vi "Destroy Events.vi"(8 "error in (no error)":errorcluster, 11 "NI Force Task in":refnum<class "NI Force Task.lvclass">) -> (0 "error out":errorcluster, 3 "NI Force Task out":refnum<class "NI Force Task.lvclass">)   [LabVIEW 2020, in "NI Force Task.lvlib" / "NI Force Task.lvclass"]
uses:
  NI Force Task.lvclass
  C:/Program Files/National Instruments/LabVIEW 2020/vi.lib/ActorFramework/Actor/Actor.lvclass
  <vilib>/ActorFramework/Actor/Actor.lvclass/Actor.ctl
  NI Force Task.lvclass/NI Force Task.ctl
  GUI Interface Messages/End Preview Msg/End Preview Msg.lvclass/End Preview Msg.ctl
  <vilib>/ActorFramework/Message Enqueuer/Message Enqueuer.lvclass/Message Enqueuer.ctl
  <vilib>/ActorFramework/Message Enqueuer/Enqueue.vi
  GUI Interface Messages/End Preview Msg/End Preview Msg.lvclass
  C:/Program Files/National Instruments/LabVIEW 2020/vi.lib/ActorFramework/Message/Message.lvclass
  <vilib>/ActorFramework/Stop Msg/Stop Msg.lvclass
  <vilib>/ActorFramework/Message Priority Queue/Priority Enqueue.vi
  <vilib>/ActorFramework/Actor/Actor.lvclass
panel:
  out "error out 2":errorcluster
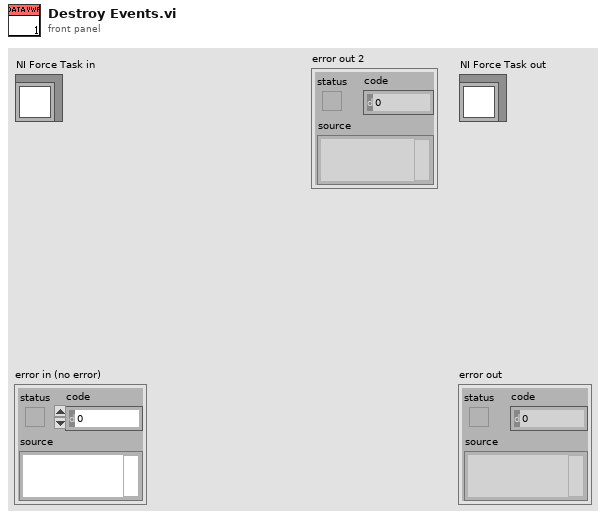
[diagram p1: front panel]
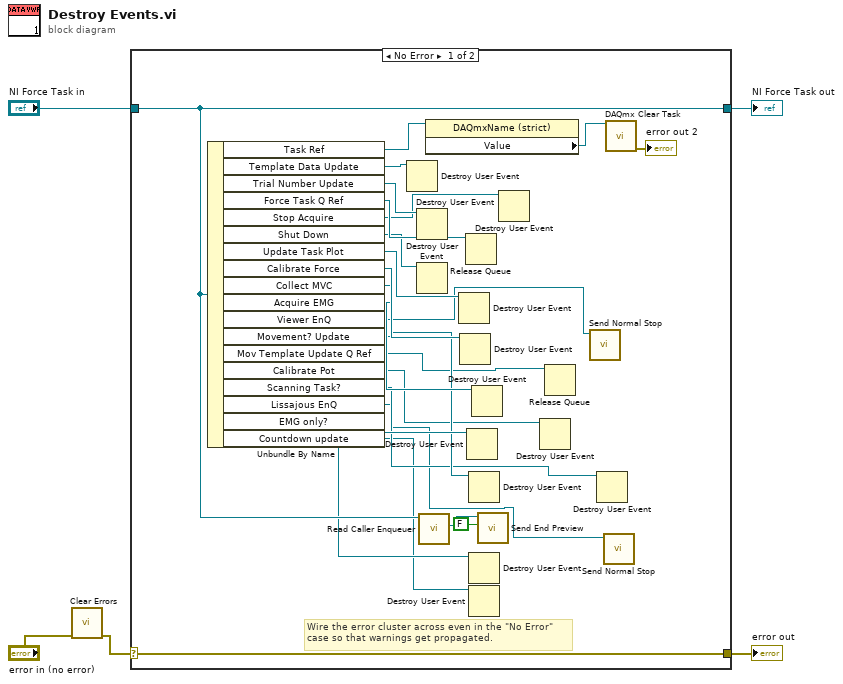
[diagram p0: block diagram]
diagram:
  n1 = call <vilib>:"Clear Errors.vi"("error in (no error)"="error in (no error)") -> ("error out"=w1:errorcluster)  [unwired: 5 in, 1 out]
  n2 = case shown="No Error" w1 {
    selector: w1 -> [w29 w31]
    tunnel: [w29 w31] -> w5
    tunnel: [w15 w30] -> w3
    tunnel: "NI Force Task in" -> [w15 w30]
    frame No Error {
      # "Wire the error cluster across even in the \"No Error\"\ncase so that warnings get propagated."
      n3 = Unbundle By Name(w15) -> ("Task Ref"=w22:refnum<vi>, "Template Data Update"=w28:refnum<user-event>, "Trial Number Update"=w27:refnum<user-event>, "Force Task Q Ref"=w26:refnum<queue>, "Stop Acquire"=w25:refnum<user-event>, "Shut Down"=w24:refnum<user-event>, "Update Task Plot"=w20:refnum<user-event>, "Calibrate Force"=w19:refnum<user-event>, "Collect MVC"=w18:refnum<user-event>, "Acquire EMG"=w17:refnum<user-event>, "Viewer EnQ"=w13:refnum<class "Message Enqueuer.lvclass">, "Movement? Update"=w12:refnum<user-event>, "Mov Template Update Q Ref"=w11:refnum<queue>, "Calibrate Pot"=w10:refnum<user-event>, "Scanning Task?"=w9:refnum<user-event>, "Lissajous EnQ"=w8:refnum<class "Message Enqueuer.lvclass">, "EMG only?"=w7:refnum<user-event>, "Countdown update"=w6:refnum<user-event>)
      n4 = Destroy User Event(user event=w28) -> ()  [unwired: 1 in, 1 out]
      n5 = Destroy User Event(user event=w27) -> ()  [unwired: 1 in, 1 out]
      n6 = Destroy User Event(user event=w24) -> ()  [unwired: 1 in, 1 out]
      n7 = call <vilib>:"Read Caller Enqueuer.vi"("Actor"=w15) -> ("Caller Enqueuer"=w16:refnum<class "Message Enqueuer.lvclass">)  [unwired: 10 in]
      n8 = property class="DAQmxName (strict)"(reference=w22) -> ("Value"=w21:refnum<k21>)  [unwired: 1 in, 2 out]
      n9 = Destroy User Event(user event=w20) -> ()  [unwired: 1 in, 1 out]
      n10 = Destroy User Event(user event=w19) -> ()  [unwired: 1 in, 1 out]
      n11 = Release Queue(queue=w26) -> ()  [unwired: 2 in, 3 out]
      n12 = Destroy User Event(user event=w17) -> ()  [unwired: 1 in, 1 out]
      n13 = Destroy User Event(user event=w12) -> ()  [unwired: 1 in, 1 out]
      n14 = Destroy User Event(user event=w7) -> ()  [unwired: 1 in, 1 out]
      n15 = Destroy User Event(user event=w6) -> ()  [unwired: 1 in, 1 out]
      n16 = Destroy User Event(user event=w18) -> ()  [unwired: 1 in, 1 out]
      n17 = call "Send End Preview.vi"("Preview"=FALSE, "Message Enqueuer"=w16) -> ()  [unwired: 8 in, 2 out]
      n18 = Destroy User Event(user event=w25) -> ()  [unwired: 1 in, 1 out]
      n19 = Destroy User Event(user event=w10) -> ()  [unwired: 1 in, 1 out]
      n20 = Release Queue(queue=w11) -> ()  [unwired: 2 in, 3 out]
      n21 = call <vilib>:"Send Normal Stop.vi"("Message Enqueuer"=w13) -> ()  [unwired: 10 in, 1 out]
      n22 = Destroy User Event(user event=w9) -> ()  [unwired: 1 in, 1 out]
      n23 = call <vilib>:"Send Normal Stop.vi"("Message Enqueuer"=w8) -> ()  [unwired: 10 in, 1 out]
      n24 = call <vilib>:"DAQmx Clear Task.vi"("task in"=w21) -> ("error out"=→"error out 2":errorcluster)  [unwired: 14 in]
    }
    frame Error {
    }
  }
  "error out" <- w5
  "NI Force Task out" <- w3
